vi "acquireData.vi"() -> ()   [LabVIEW 2015]
panel:
  in  "zInc(mm)":dbl
  in  "Base path":path=path "C:/Users/sims01/Desktop/dataAcq"
  in  "no z steps":i32=2
  in  "initPosZ(mm)":dbl
  in  "642 nm filter":T1(ring)=enum."665/LP [Cy5]"
  in  "561 nm filter":T1(ring)=enum."605/70 [Cy3]"
  in  "488 nm filter":T1(ring)=enum."525/50 [FITC]"
  in  "405 nm filter":T1(ring)
  in  "Filter wheel init":cluster{"FW Handle":u32, "init?":i16}
  in  "Z stage":T2
  in  "XY stage":T3
  in  "sCMOS init":cluster{"init":i16, "sCMOS handle":u32}
  in  "405 nm (aq)":bool=TRUE
  in  "488 nm (aq)":bool=TRUE
  in  "561 nm (aq)":bool=TRUE
  in  "642 nm (aq)":bool=TRUE
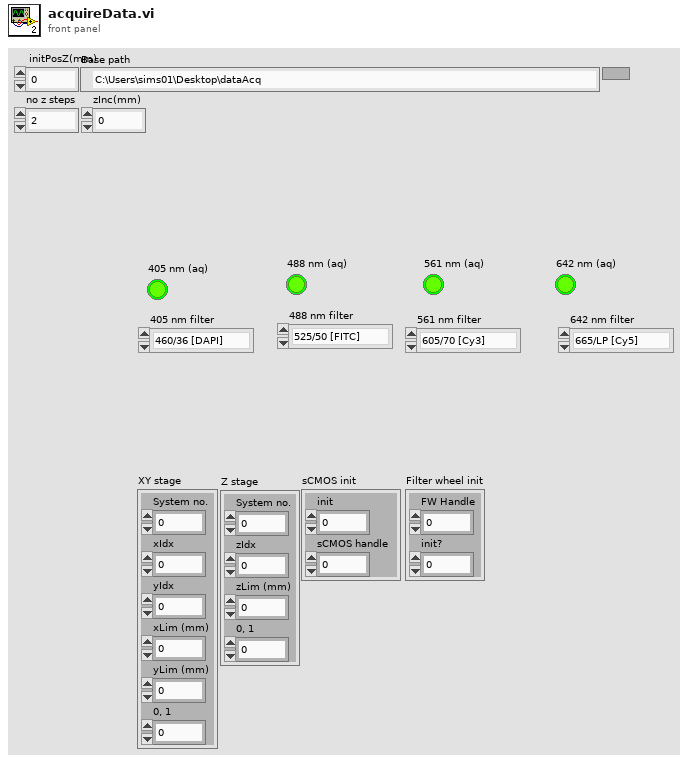
[diagram p1: front panel]
types:
  T1 = enum16{"460/36 [DAPI]", "525/50 [FITC]", "605/70 [Cy3]", "665/LP [Cy5]", "Empty-1", "Empty-2"}
  T2 = cluster{"System no.":i32, "zIdx":i32, "zLim (mm)":dbl, "0, 1":i16}
  T3 = cluster{"System no.":i32, "xIdx":i32, "yIdx":i32, "xLim (mm)":dbl, "yLim (mm)":dbl, "0, 1":i16}
  T4 = enum16{"460/36 [DAPI]", "525/50 [FITC]", "605/70 [Cy3]", "665/LP [Cy5]", "Empty-1", "Empty-2"}[]
  T5 = cluster{"Component ID":string, "COM Port":refnum<visa-resource-name>, "Type ":enum16{"omicronLuxX", "coherentObis"}, "init":i16}[]
  T6 = cluster{"Component ID":string, "COM Port":refnum<visa-resource-name>, "Type ":enum16{"omicronLuxX", "coherentObis"}, "init":i16}
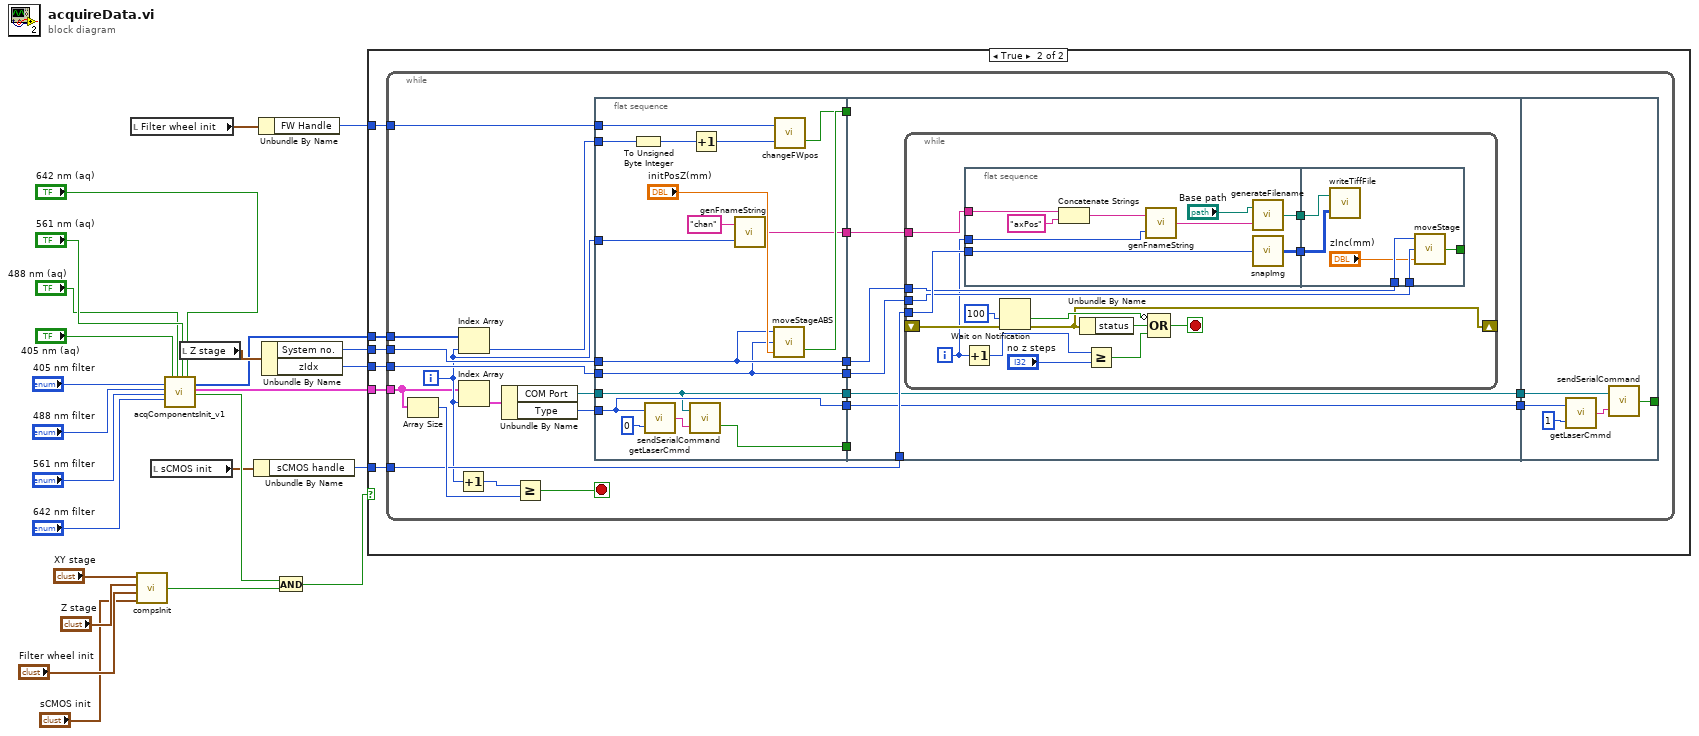
[diagram p0: block diagram]
diagram:
  n1 = local read "Filter wheel init"() -> (w9:cluster{"FW Handle":u32, "init?":i16})
  n2 = call "compsInit.vi"("XY stage"="sCMOS init", "Filter wheel init"="Filter wheel init", "sCMOS init"="Z stage", "Z stage"="XY stage") -> ("allComponentsInit?"=w15:bool)
  n3 = local read "sCMOS init"() -> (w2:cluster{"init":i16, "sCMOS handle":u32})
  n4 = call "acqComponentsInit_v1.vi"("405 nm filter"="405 nm filter", "488 nm filter"="488 nm filter", "561 nm filter"="561 nm filter", "642 nm filter"="642 nm filter", "405 nm (aq)"="405 nm (aq)", "488 nm (aq)"="488 nm (aq)", "561 nm (aq)"="561 nm (aq)", "642 nm (aq)"="642 nm (aq)") -> ("Initialized filters"=w4:T4, "initializedLasers"=w3:T5, "correctCompInit?"=w20:bool)  [unwired: 9 in]
  n5 = local read "Z stage"() -> (w7:T2)
  n6 = Unbundle By Name(w2) -> ("sCMOS handle"=w1:u32)
  n7 = Unbundle By Name(w9) -> ("FW Handle"=w8:u32)
  n8 = Unbundle By Name(w7) -> ("System no."=w6:i32, "zIdx"=w5:i32)
  n9 = And(x=w20, y=w15) -> (x .and. y?=w10:bool)
  n10 = case shown="True" w10 {
    tunnel: w8 -> [_ w30]
    tunnel: w6 -> [_ w29]
    tunnel: w5 -> [_ w28]
    tunnel: w4 -> [_ w27]
    tunnel: w3 -> [_ w26]
    tunnel: w1 -> [_ w25]
    frame False {
    }
    frame True {
      n11 = while {
        tunnel: w30 -> [w49]
        tunnel: w29 -> [w48]
        tunnel: w28 -> [w47]
        tunnel: w27 -> [w46]
        tunnel: w26 -> [w35]
        tunnel: w25 -> [w41]
        i -> [w38]
        stop <- w52 stop-if-true
        n12 = Array Size(array=w35) -> (size(s)=w54:i32)
        n13 = Increment(x=w38) -> (x+1=w53:i32)
        n14 = Index Array(array=w46, index=w38) -> (element=w45:T1)
        n15 = Index Array(array=w35, index=w38) -> (element=w44:T6)
        n16 = Unbundle By Name(w44) -> ("COM Port"=w50:refnum<visa-resource-name>, "Type"=w51:enum16{"omicronLuxX", "coherentObis"})
        n17 = Greater Or Equal?(x=w53, y=w54) -> (x >= y?=w52:bool)
        n18 = flat-sequence {
          tunnel: w51 -> [w56]
          tunnel: w50 -> [w55]
          tunnel: w49 -> [w66]
          tunnel: w48 -> [w62]
          tunnel: w47 -> [w61]
          tunnel: w45 -> [w65]
          tunnel: [w67] -> w43
          tunnel: [w63] -> w42
          tunnel: [w62] -> w40
          tunnel: [w61] -> w39
          tunnel: w38 -> [w59]
          tunnel: [w58] -> w37
          tunnel: [w57] -> w36
          tunnel: [w56] -> w34
          tunnel: [w55] -> w32
          tunnel: w43 -> [_]
          tunnel: w42 -> [_]
          tunnel: w41 -> [w77]
          tunnel: w40 -> [w76]
          tunnel: w39 -> [w75]
          tunnel: w37 -> [w74]
          tunnel: w36 -> [_]
          tunnel: w34 -> [w73]
          tunnel: [w73] -> w33
          tunnel: w32 -> [w72]
          tunnel: [w72] -> w31
          tunnel: w33 -> [w111]
          tunnel: w31 -> [w110]
          tunnel: [w109] -> _
          frame #0 {
            n19 = To Unsigned Byte Integer(number=w65) -> (unsigned 8bit integer=w69:u8)
            n20 = call "getLaserCmmd.vi"("Cmmd index"=0, "Laser type"=w56) -> ("Laser command"=w70:string)
            n21 = call "sendSerialCommand.vi"("Cmmd"=w70, "input COM Port"=w55) -> ("data written to port?"=w67:bool)
            n22 = Increment(x=w69) -> (x+1=w68:u8)
            n23 = call "genFnameString.vi"("Idx"=w59, "str"="chan") -> ("fName"=w58:string)
            n24 = call "moveStageABS.vi"("absolute pos (mm)"="initPosZ(mm)", "axisIdx"=w61, "System no."=w62) -> ("Stopped"=w63:bool)
            n25 = call "changeFWpos.vi"("FW pos"=w68, "FWhandle"=w66) -> ("fwPosChanged"=w57:bool)
          }
          frame #1 {
            n26 = while {
              shift-right: [w86] -> _
              shift-left: _ -> [w87]
              tunnel: w77 -> [w82]
              tunnel: w76 -> [w81]
              tunnel: w75 -> [w80]
              tunnel: w74 -> [w79]
              i -> [w78]
              stop <- w85 stop-if-true
              n27 = Increment(x=w78) -> (x+1=w92:i32)
              n28 = flat-sequence {
                tunnel: [w100] -> w84
                tunnel: [w102] -> w83
                tunnel: w82 -> [w101]
                tunnel: w79 -> [w99]
                tunnel: w78 -> [w95]
                tunnel: w84 -> [w108]
                tunnel: w83 -> [w107]
                tunnel: w81 -> [w106]
                tunnel: w80 -> [w105]
                tunnel: [w104] -> _
                frame #0 {
                  n29 = Concatenate Strings(w99, "axPos") -> (w98:string)
                  n30 = call "genFnameString.vi"("Idx"=w95, "str"=w98) -> ("fName"=w97:string)
                  n31 = call "generateFilename.vi"("Filename"=w97, "Base path"="Base path") -> ("Appended path"=w100:path)
                  n32 = call "snapImg.vi"("Handle in"=w101) -> ("16bitImgFile"=w102:u16[][])
                }
                frame #1 {
                  n33 = call "writeTiffFile.vi"("Image Pixels (U16)"=w107, "File Path"=w108) -> ()
                  n34 = call "moveStage.vi"("inc (mm)"="zInc(mm)", "axisIdx"=w105, "System no."=w106) -> ("Stopped"=w104:bool)
                }
              }
              n35 = Wait on Notification(timeout in ms (-1)=100, error in (no error)=w87) -> (timed out?=w89:bool, error out=w86:errorcluster)  [unwired: 2 in, 2 out]
              n36 = Unbundle By Name(w86) -> ("status"=w90:bool)
              n37 = Greater Or Equal?(x=w92, y="no z steps") -> (x >= y?=w91:bool)
              n38 = Compound Arithmetic op=OR(invert w89, w90, w91) -> (w85:bool)
            }
          }
          frame #2 {
            n39 = call "getLaserCmmd.vi"("Cmmd index"=1, "Laser type"=w111) -> ("Laser command"=w113:string)
            n40 = call "sendSerialCommand.vi"("Cmmd"=w113, "input COM Port"=w110) -> ("data written to port?"=w109:bool)
          }
        }
      }
    }
  }
